vi "36-sub-palindrome-base-2-check.vi"(1 "Number":u64) -> (0 "Number is Palindrome in Base 2?":bool)   [LabVIEW 2021]
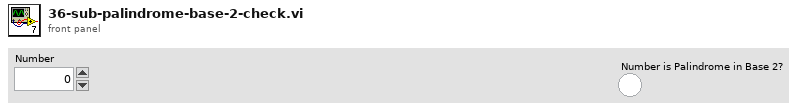
[diagram p1: front panel]
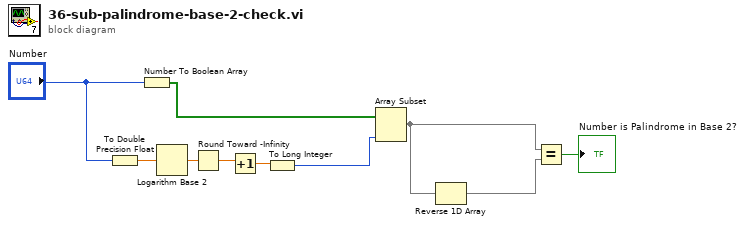
[diagram p0: block diagram]
diagram:
  n1 = To Double Precision Float(number="Number") -> (double precision float=w9:dbl)
  n2 = Number To Boolean Array(number="Number") -> (Boolean array=w5:bool[])
  n3 = Logarithm Base 2(1:w9) -> (0:w8:dbl)
  n4 = Round Toward -Infinity(1:w8) -> (0:w7:dbl)
  n5 = Increment(x=w7) -> (x+1=w6:dbl)
  n6 = To Long Integer(number=w6) -> (32bit integer=w4:i32)
  n7 = Array Subset(array=w5, length=w4) -> (w3:bool[])  [unwired: 1 in]
  n8 = Reverse 1D Array(array=w3) -> (reversed array=w2:bool[])
  n9 = Equal?(x=w3, y=w2) -> (x = y?=→"Number is Palindrome in Base 2?":bool)
